vi "Build_Filename_with_Date_Time.vi"(9 "File Extension (.csv)":string, 10 "Item Prefix":string, 11 "Folder for Data Captures":path) -> (3 "File Path Output":string)   [LabVIEW 2021]
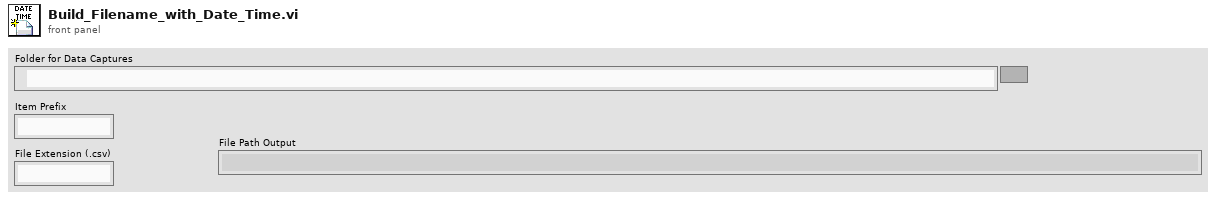
[diagram p1: front panel]
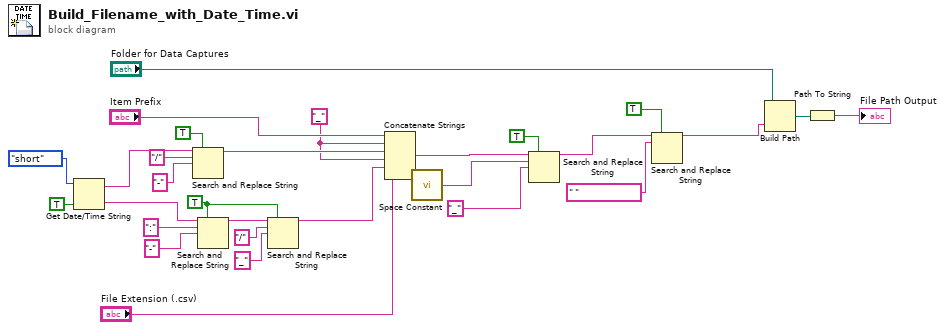
[diagram p0: block diagram]
diagram:
  w15 = "_" ("replace string (\"\")")
  w21 = TRUE ("replace all? (F)")
  n1 = Get Date/Time String(date format (0)=enum16{"short", "long", "abbreviated"}."short", want seconds? (F)=TRUE) -> (date string=w9:string, time string=w26:string)  [unwired: 1 in]
  n2 = Search and Replace String(replace all?=TRUE ("replace all? (F)"), input string=w9, search string="/" ("replace string (\"\")"), replace string="-" ("replace string (\"\")")) -> (result string=w16:string)  [unwired: 4 in, 3 out]
  n3 = Search and Replace String(replace all?=w21, input string=w26, search string=":" ("replace string (\"\")"), replace string="-" ("replace string (\"\")")) -> (result string=w23:string)  [unwired: 4 in, 3 out]
  n4 = Search and Replace String(replace all?=w21, input string=w23, search string="/" ("replace string (\"\")"), replace string="_" ("replace string (\"\")")) -> (result string=w22:string)  [unwired: 4 in, 3 out]
  n5 = Concatenate Strings("Item Prefix", w15, w16, w15, w22, "File Extension (.csv)") -> (w14:string)
  n6 = call <vilib>:"Space Constant.vi"() -> ("String"=w12:string)
  n7 = Search and Replace String(replace all?=TRUE ("replace all? (F)"), input string=w14, search string=w12, replace string="_" ("replace string (\"\")")) -> (result string=w4:string)  [unwired: 4 in, 3 out]
  n8 = Search and Replace String(replace all?=TRUE ("replace all? (F)"), input string=w4, search string=" ") -> (result string=w3:string)  [unwired: 5 in, 3 out]
  n9 = Build Path(base path="Folder for Data Captures", name or relative path=w3) -> (appended path=w6:path)
  n10 = Path To String(path=w6) -> (string=→"File Path Output":string)
